vi "Init.vi"(4 "False":refnum<class "CConfig Query.lvclass">, 6 "True":refnum<class "CConfig Query.lvclass">, 8 "error in (no error)":errorcluster, 10 "If":refnum<class "CConfig Query.lvclass">) -> (0 "error out":errorcluster, 3 "Find First Query out":refnum<class "If Query.lvclass">)   [LabVIEW 2013, in "If Query.lvclass"]
doc: "Copyright 2018, Carya Automatisering, Wiebe Walstra."
uses:
  If Query.lvclass
  CConfig Query.lvclass
  If Query.lvclass/If Query.ctl
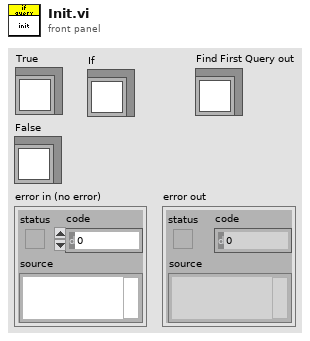
[diagram p1: front panel]
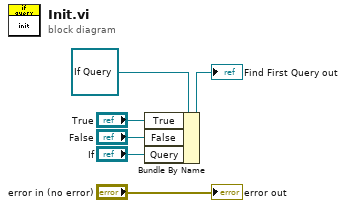
[diagram p0: block diagram]
diagram:
  n1 = Bundle By Name(cluster=refnum<class "If Query.lvclass"> refnum ("Find First Query in"), "True"="True", "False"="False", "Query"="If") -> (→"Find First Query out":refnum<class "If Query.lvclass">)
  "error out" <- "error in (no error)"
